vi "Create Simple QA Agent State Machine.vi"() -> (3 "return value":i16)   [LabVIEW 2020]
panel:
  # "Creating LabVIEW LLM Simple QA Agent State Machine"
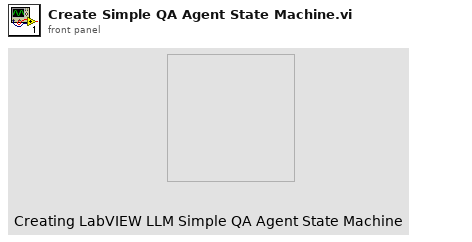
[diagram p1: front panel]
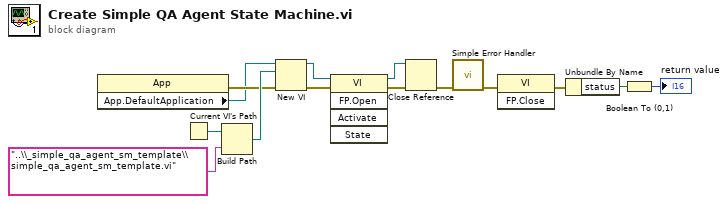
[diagram p0: block diagram]
diagram:
  n1 = property class="App"() -> (error out=w2:errorcluster, "App.DefaultApplication"=w1:refnum<vi>)  [unwired: 2 in, 1 out]
  n2 = Current VI's Path() -> (path=w9:path)
  n3 = Build Path(base path=w9, name or relative path="..\\_simple_qa_agent_sm_template\\simple_qa_agent_sm_template.vi") -> (appended path=w7:path)
  n4 = New VI(8:w2, 10:w7, 11:w1) -> (0:w13:errorcluster, 3:w14:refnum<vi>)  [unwired: 4 out]
  n5 = invoke class="VI" method="FP.Open"(reference=w14, error in=w13) -> (reference out=w11:refnum<vi>, error out=w10:errorcluster)  [unwired: 3 in, 3 out]
  n6 = Close Reference(reference=w11, error in (no error)=w10) -> (error out=w12:errorcluster)
  n7 = call <vilib>:"Simple Error Handler.vi"("error in (no error)"=w12) -> ("error out"=w6:errorcluster)  [unwired: 1 in, 7 out]
  n8 = invoke class="VI" method="FP.Close"(error in=w6) -> (error out=w5:errorcluster)  [unwired: 2 in, 2 out]
  n9 = Unbundle By Name(w5) -> ("status"=w4:bool)
  n10 = Boolean To (0,1)(Boolean=w4) -> (0, 1=→"return value":i16)
